vi "Enum Simulator 2015.vi"() -> ()   [LabVIEW 2014]
uses:
  Common Code/Elevator Mode.ctl
panel:
  out "Mode":T1
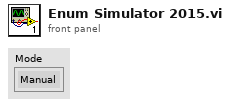
[diagram p1: front panel]
types:
  T1 = typedef "Elevator Mode.ctl" = enum16{"Manual", "Safe", "Auto"}
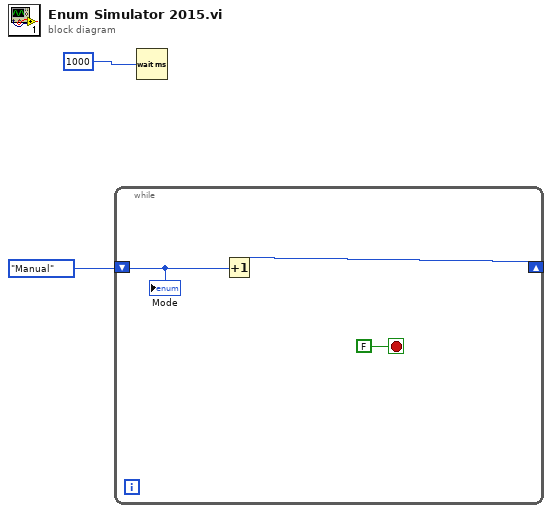
[diagram p0: block diagram]
diagram:
  n1 = while {
    shift-right: [w3] -> _
    shift-left: Elevator_Mode."Manual" ("Mode") -> [w5]
    stop <- FALSE stop-if-true
    n2 = Increment(x=w5) -> (x+1=w3:T1)
    "Mode" <- w5
  }
  n3 = Wait (ms)(milliseconds to wait=u32 1000) -> ()  [unwired: 1 out]
